vi "Read Single Gate in SS2 Data Group.vi"(5 "SS2 8-bit Frame Selection":T1 caption="SS2 Frame Selection", 6 "Gate Idx":i32, 7 "Bitness":i32, 8 "error in (no error)":errorcluster, 9 "Pixel Y":i32, 10 "Pixel X":i32, 11 "group in":T2 format="%.0x") -> (0 "error out":errorcluster, 1 "DAQ Time":dbl[unit], 2 "Data":u16[](array[numeric]), 3 "group out":T2 format="%.0x", 4 "# 8-bit frames":i32)   [LabVIEW 2021, in "SwissSPAD.lvlib"]
uses:
  SwissSPAD.lvlib
  <vilib>/addons/h5labview2/base/hid_t.ctl
  SwissSPAD 8-bit Frames Read.ctl
  SS2 Data List.ctl
  <vilib>/addons/h5labview2/base/lib_path.vi
  <vilib>/addons/h5labview2/base/H5Equery.vi
  <vilib>/Utility/error.llb/Error Cluster From Error Code.vi
  <vilib>/addons/h5labview2/dataset/H5Dread.llb/H5Dread.xnode
  <vilib>/ErrorRing/Error Ring.xnode
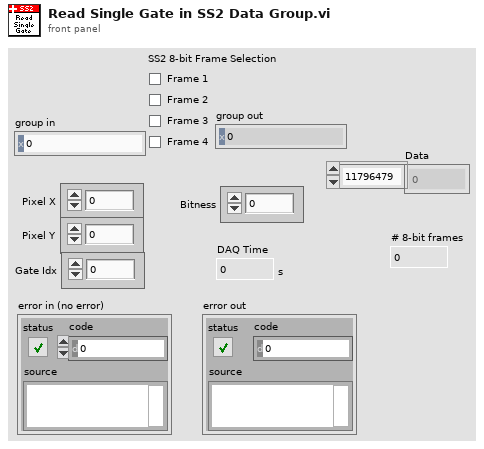
[diagram p1: front panel]
types:
  T1 = typedef "SwissSPAD.lvlib/SwissSPAD 8-bit Frames Read.ctl" = cluster{"Frame 1":bool, "Frame 2":bool, "Frame 3":bool, "Frame 4":bool}
  T2 = typedef "hid_t.ctl" = i64
  T3 = typedef "SwissSPAD.lvlib/SS2 Data List.ctl" = enum16{"daq_time_s", "data"}
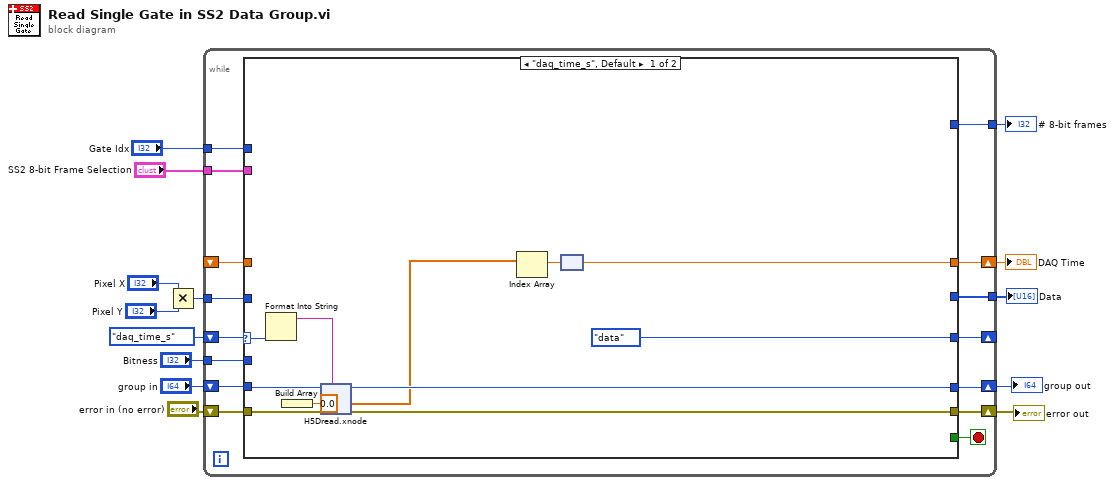
[diagram p0: block diagram]
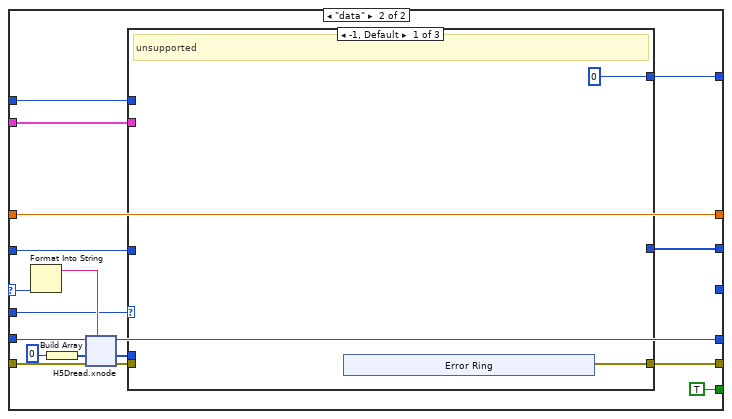
[diagram p2: hidden frame]
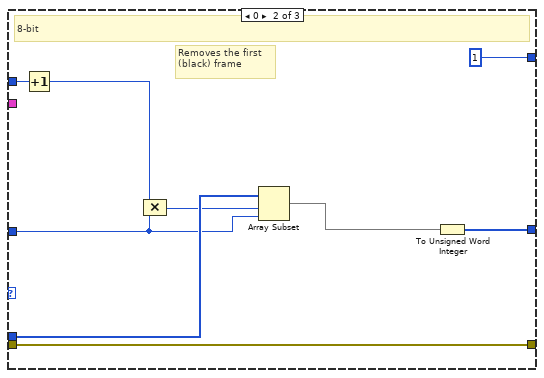
[diagram p3: hidden frame]
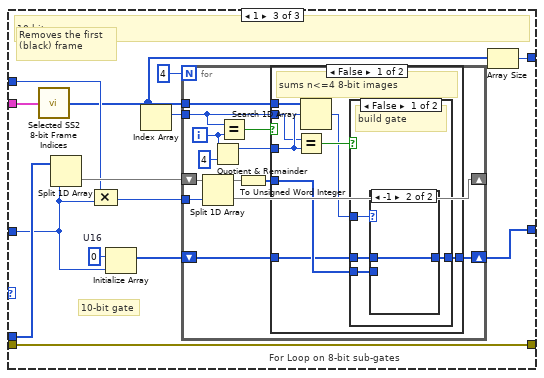
[diagram p4: hidden frame]
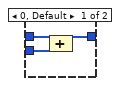
[diagram p5: hidden frame]
diagram:
  n1 = Multiply(x="Pixel X", y="Pixel Y") -> (x*y=w8:i32)
  n2 = while {
    shift-right: [w25] -> w13
    shift-left: "error in (no error)" -> [w26]
    shift-right: [w27] -> w11
    shift-left: "group in" -> [w28]
    shift-right: [w23] -> _
    shift-left: SS2_Data_List."daq_time_s" ("SS2 Data") -> [w29]
    shift-right: [w24] -> w9
    shift-left: _ -> [w22]
    tunnel: w8 -> [w20]
    tunnel: "Gate Idx" -> [w19]
    tunnel: "Bitness" -> [w18]
    tunnel: [w17] -> w5
    tunnel: "SS2 8-bit Frame Selection" -> [w16]
    tunnel: [w15] -> w1
    stop <- w21 stop-if-true
    n3 = case shown="\"daq_time_s\", Default" w29 {
      selector: w29 -> [w40 w73]
      tunnel: w28 -> [w39 w72]
      tunnel: [w38 w71] -> w27
      tunnel: w26 -> [w37 w70]
      tunnel: [w36 w58] -> w25
      tunnel: [w31 w67] -> w24
      tunnel: [SS2_Data_List."data" ("SS2 Data") _] -> w23
      tunnel: w22 -> [_ w67]
      tunnel: [_ TRUE] -> w21
      tunnel: w20 -> [_ w63]
      tunnel: w19 -> [_ w64]
      tunnel: w18 -> [_ w62]
      tunnel: [_ w61] -> w17
      tunnel: w16 -> [_ w60]
      tunnel: [_ w57] -> w15
      frame "daq_time_s", Default {
        n4 = Format Into String(w40) -> (resulting string=w41:string)  [unwired: 3 in, 1 out]
        n5 = Build Array(0.0) -> (w33:dbl[])
        n6 = xnode "H5Dread.xnode"("dataset name (this)"=w41, "error in (no error)"=w37, "default"=w33, "ref in"=w39) -> ("error out"=w36:errorcluster, "data"=w34:dbl[], "ref out"=w38:i64)  [unwired: 2 in, 1 out]
        n7 = Index Array(array=w34) -> (element=w32:dbl)  [unwired: 1 in]
        n8 = node(w32) -> (w31:dbl[unit])
      }
      frame "data" {
        n9 = Format Into String(w73) -> (resulting string=w74:string)  [unwired: 3 in, 1 out]
        n10 = Build Array(u8 0) -> (w68:u8[])
        n11 = xnode "H5Dread.xnode"("dataset name (this)"=w74, "error in (no error)"=w70, "default"=w68, "ref in"=w72) -> ("error out"=w59:errorcluster, "data"=w65:u8[], "ref out"=w71:T2)  [unwired: 2 in, 1 out]
        n12 = case shown="-1, Default" w62 {
          tunnel: w65 -> [_ w101 w118]
          tunnel: w64 -> [_ w100 w109]
          tunnel: w63 -> [_ w98 w110]
          tunnel: [_ w104 w105] -> w61
          tunnel: w60 -> [_ _ w114]
          tunnel: w59 -> [_ w103 w112]
          tunnel: [w91 w103 w112] -> w58
          tunnel: [0 1 w107] -> w57
          frame -1, Default {
            # "unsupported"
            n13 = xnode "Error Ring"() -> ("error out"=w91:errorcluster)
          }
          frame 0 {
            # "Removes the first (black) frame"
            # "8-bit"
            n14 = Increment(x=w100) -> (x+1=w96:i32)
            n15 = Compound Arithmetic op=MULTIPLY(w96, w98) -> (w99:i32)
            n16 = Array Subset(array=w101, index=w99, length=w98) -> (w97:u8[])
            n17 = To Unsigned Word Integer(number=w97) -> (unsigned 16bit integer=w104:u16[])
          }
          frame 1 {
            w117 = u16 0  # U16
            # "Removes the first (black) frame"
            # "10-bit gate"
            # "10-bit"
            n18 = call "Selected SS2 8-bit Frame Indices.vi"("SS2 8-bit Frame Selection"=w114) -> ("Selected 8-bit Frame Indices"=w106:i32[])
            n19 = Split 1D Array(array=w118, index=w110) -> (second subarray=w115:u8[])  [unwired: 1 out]
            n20 = Compound Arithmetic op=MULTIPLY(w109, w110) -> (w108:i32)
            n21 = Initialize Array(w117, w110) -> (w116:u16[])
            n22 = Index Array(array=w106) -> (element=w113:i32)  [unwired: 1 in]
            n23 = for "For Loop on 8-bit sub-gates" {
              N: 4 ("value") -> [_]
              shift-right: [w126] -> _
              shift-left: w115 -> [w131]
              tunnel: w108 -> [w130]
              shift-right: [w127] -> w105
              shift-left: w116 -> [w128]
              tunnel: w106 -> [w120]
              tunnel: w113 -> [w119]
              i -> [w122]
              n24 = Split 1D Array(array=w131, index=w130) -> (first subarray=w129:u8[], second subarray=w126:u8[])
              n25 = Quotient & Remainder(x=w122, y=4) -> (x-y*floor(x/y)=w121:i32)  [unwired: 1 out]
              n26 = Equal?(x=w119, y=w122) -> (x = y?=w123:bool)
              n27 = To Unsigned Word Integer(number=w129) -> (unsigned 16bit integer=w125:u16[])
              n28 = case shown="False" w123 {
                tunnel: w125 -> [w139 w149]
                tunnel: w128 -> [w138 _]
                tunnel: [w137 w149] -> w127
                tunnel: w121 -> [w135 _]
                tunnel: w120 -> [w136 _]
                tunnel: w119 -> [w134 _]
                frame False {
                  # "sums n<=4 8-bit images"
                  n29 = Equal?(x=w134, y=w135) -> (x = y?=w133:bool)
                  n30 = Search 1D Array(1D array=w136, element=w135) -> (index of element=w132:i32)  [unwired: 1 in]
                  n31 = case shown="False" w133 {
                    tunnel: w139 -> [w141 w148]
                    tunnel: w138 -> [w142 _]
                    tunnel: [w143 w148] -> w137
                    tunnel: w132 -> [w140 _]
                    frame False {
                      # "build gate"
                      n32 = case shown="-1" w140 {
                        tunnel: [w146 w147] -> w143
                        tunnel: w142 -> [w145 w147]
                        tunnel: w141 -> [w144 _]
                        frame 0, Default {
                          n33 = Compound Arithmetic op=ADD(w145, w144) -> (w146:u16[])
                        }
                        frame -1 {
                        }
                      }
                    }
                    frame True {
                      # "new gate"
                    }
                  }
                }
                frame True {
                  # "First selected 8-bit frame"
                }
              }
            }
            n34 = Array Size(array=w106) -> (size(s)=w107:i32)
          }
        }
      }
    }
  }
  "group out" <- w11
  "error out" <- w13
  "DAQ Time" <- w9
  "Data" <- w5
  "# 8-bit frames" <- w1
